vi "Perform Measurement - WaveformMode.vi"(8 "error in":errorcluster, 10 "Measure Call Context in":refnum<class "Measure Call Context.lvclass">, 11 "measurement configuration":T2={"Mode of operation"=enum."Power on the DUT", "Source voltage/current gain bandwidths"=[], "Source voltage/current compensation frequencies"=[], "Source voltage/current pole-zero ratios"=[], "Load voltage/current gain bandwidths"=[], "Load voltage/current compensation frequencies"=[], "Load voltage/current pole-zero ratios"=[], "Source enable/disable"=FALSE, "Load enable/disable"=FALSE, "Power ON/Source resource names"=[], "Load resource names"=[], "Power ON/Source voltage/current setpoints"=[], "Source source delays"=[], "Load voltage/current setpoints"=[], "Load source delays"=[], "Power ON/Source system configuration"=enum."Series", "Power ON/Source output function"=0, "Source voltage/current level range"=0.0, "Power ON/Source sense"=0, "Source limit symmetry"=enum."Symmetric", "Power ON/Source current/voltage limit range"=0.0, "Source current/voltage limit low"=0.0, "Source current/voltage limit high"=0.0, "Source aperture time"=0.0, "Source transient response"=0, "Load device voltage/current rating"=10.0, "Load system configuration"=enum."Series", "Load output function"=0, "Load voltage/current level range"=0.0, "Load sense"=0, "Load limit symmetry"=enum."Symmetric", "Load current/voltage limit range"=0.0, "Load current/voltage limit low"=0.0, "Load current/voltage limit high"=0.0, "Load aperture time"=0.0, "Load transient response"=0, "Measurement timeout"=1.0} {"Measurement timeout" format="%.3p"; "Load voltage/current setpoints" format="%#_6p"; "Load output function" items=["DC Voltage"=1006, "DC Current"=1007, "Pulse Voltage"=1049, "Pulse Current"=1050]; "Load sense" items=["Local"=1008, "Remote"=1009]; "Load transient response" items=["Slow"=1041, "Normal"=1038, "Fast"=1039, "Custom"=1042]; "Load current/voltage limit high" format="%#_6p"; "Load current/voltage limit low" format="%#_6p"; "Load current/voltage limit range" format="%#_6p"; "Load voltage/current level range" format="%#_6p"; "Power ON/Source voltage/current setpoints" format="%#_6p"; "Power ON/Source output function" items=["DC Voltage"=1006, "DC Current"=1007, "Pulse Voltage"=1049, "Pulse Current"=1050]; "Source aperture time" format="%#_6p"; "Power ON/Source sense" items=["DC Voltage"=1006, "DC Current"=1007, "Pulse Voltage"=1049, "Pulse Current"=1050]; "Source transient response" items=["Slow"=1041, "Normal"=1038, "Fast"=1039, "Custom"=1042]; "Source current/voltage limit high" format="%#_6p"; "Source current/voltage limit low" format="%#_6p"; "Power ON/Source current/voltage limit range" format="%#_6p"; "Source voltage/current level range" format="%#_6p"}) -> (0 "error out":errorcluster, 2 "Measure Call Context out":refnum<class "Measure Call Context.lvclass">, 3 "Measurement Results":T1)   [LabVIEW 2021, in "Waveform Mode_Channel Ganging.lvlib"]
uses:
  Waveform Mode_Channel Ganging.lvlib
  shared subVIs/ctl/NIDCPower_channel_ganging - ctl - channel mode.ctl
  shared subVIs/ctl/NIDCPower_channel_ganging - ctl - ganged config.ctl
  shared subVIs/ctl/NIDCPower_channel_ganging - ctl - ganged session.ctl
  Measurement Results.ctl
  shared/Single/controls/Initialize Resource Config-Single.ctl
  shared/Ganging/controls/Initialize Resource Config-Ganging.ctl
  <instrlib>/niDCPower/nidcpower.llb/niDCPower Wait For Event - Event.ctl
  shared/Common/controls/Start and Wait for Event.ctl
  shared/Ganging/controls/Abort Single Point-Ganging.ctl
  shared/Single/controls/Abort Single Point-Single.ctl
  Controls/Waveform Mode Measurement.ctl
  shared/Single/controls/Abort Sequence-Single.ctl
  shared/Ganging/controls/Abort Sequence-Ganging.ctl
  <vilib>/Plug-In SDKs/Measurements/Measure Call Context/Measure Call Context.lvclass
  Measurement Configuration.ctl
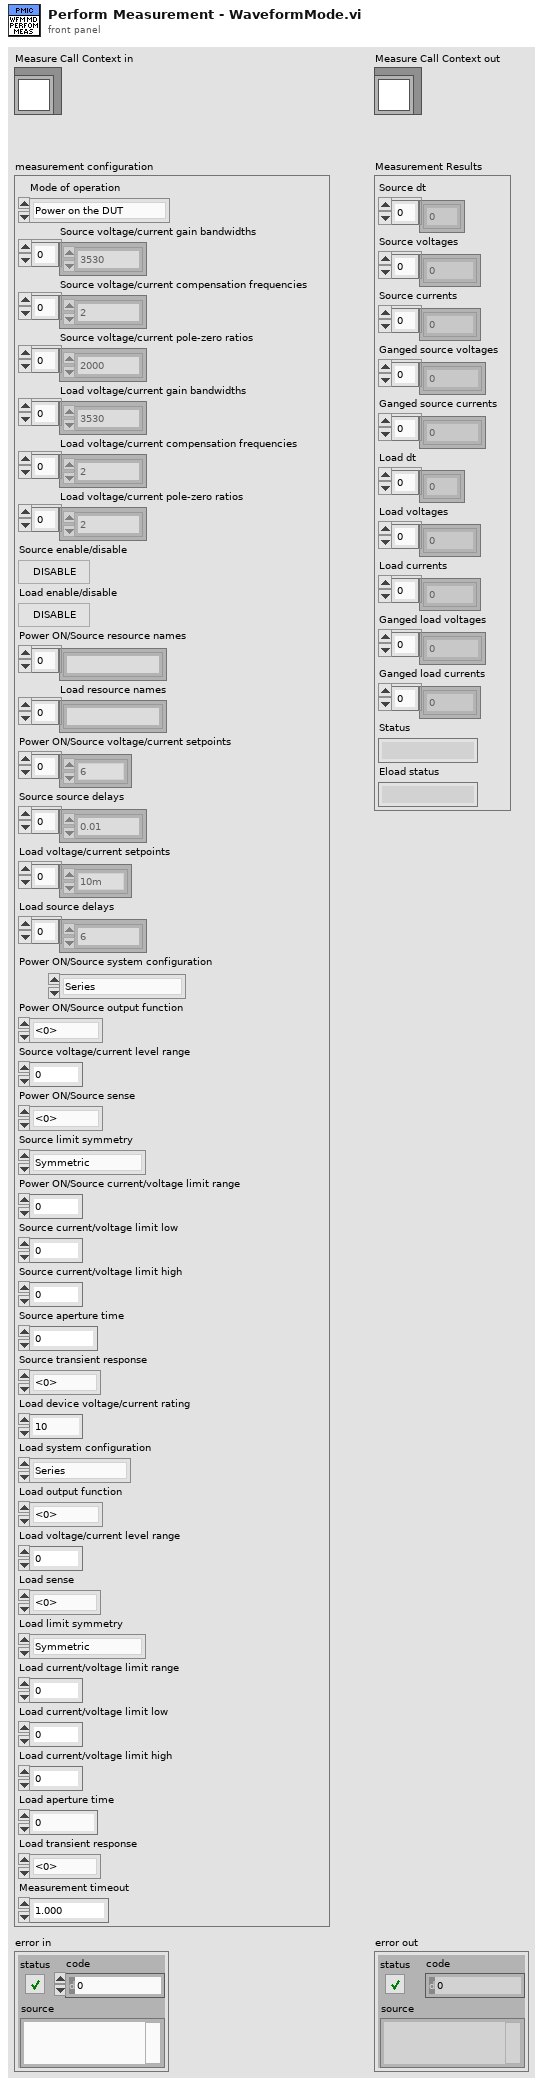
[diagram p1: front panel]
types:
  T1 = typedef "Waveform Mode_Channel Ganging.lvlib/Measurement Results.ctl" = cluster{"Source dt":dbl[], "Source voltages":dbl[], "Source currents":dbl[], "Ganged source voltages":dbl[], "Ganged source currents":dbl[], "Load dt":dbl[], "Load voltages":dbl[], "Load currents":dbl[], "Ganged load voltages":dbl[], "Ganged load currents":dbl[], "Status":string, "Eload status":string}
  T2 = typedef "Waveform Mode_Channel Ganging.lvlib/Measurement Configuration.ctl" = cluster{"Mode of operation":enum32{"Power on the DUT", "Perform measurement", "Power off the DUT"}, "Source voltage/current gain bandwidths":dbl[], "Source voltage/current compensation frequencies":dbl[], "Source voltage/current pole-zero ratios":dbl[], "Load voltage/current gain bandwidths":dbl[], "Load voltage/current compensation frequencies":dbl[], "Load voltage/current pole-zero ratios":dbl[], "Source enable/disable":bool, "Load enable/disable":bool, "Power ON/Source resource names":string[], "Load resource names":string[], "Power ON/Source voltage/current setpoints":dbl[], "Source source delays":dbl[], "Load voltage/current setpoints":dbl[], "Load source delays":dbl[], "Power ON/Source system configuration":enum32{"Series", "Parallel", "Manual"}, "Power ON/Source output function":i32, "Source voltage/current level range":dbl, "Power ON/Source sense":i32, "Source limit symmetry":enum32{"Symmetric", "Asymmetric"}, "Power ON/Source current/voltage limit range":dbl, "Source current/voltage limit low":dbl, "Source current/voltage limit high":dbl, "Source aperture time":dbl, "Source transient response":i32, "Load device voltage/current rating":dbl, "Load system configuration":enum32{"Series", "Parallel", "Manual"}, "Load output function":i32, "Load voltage/current level range":dbl, "Load sense":i32, "Load limit symmetry":enum32{"Symmetric", "Asymmetric"}, "Load current/voltage limit range":dbl, "Load current/voltage limit low":dbl, "Load current/voltage limit high":dbl, "Load aperture time":dbl, "Load transient response":i32, "Measurement timeout":dbl}
  T3 = typedef "Waveform Mode_Channel Ganging.lvlib/Waveform Mode Measurement.ctl" = cluster{"Source Ganged Session Out":T4, "Load Ganged Session Out":T4, "Source Measure Record Length":i32, "Load Measure Record Length":i32, "Source Sequence Name":string, "Load Sequence Name":string, "Source First Sequence Call":bool, "Load First Sequence Call":bool, "Measurement Results":T1, "No. of eload used":i32, "Measurement timeout":dbl, "Load Source ON/OFF":enum16{"SOURCE AND LOAD OFF", "SOURCE ON", "LOAD ON", "SOURCE AND LOAD ON"}, "Load session out":refnum<k15>, "Source session out":refnum<k15>, "Load channel name":string, "Source channel name":string, "Source ganged/single":bool, "Load ganged/single":bool, "Source Master/Single resource name":string, "Source Slave resource name":string[], "Load Master/Single resource name":string, "Load Slave resource name":string[]}
  T4 = typedef "NIDCPower_channel_ganging - ctl - ganged session.ctl" = cluster{"Ganged Config":T5, "Session List":refnum<k15>[], "Session Mode":T6[], "Channel":string[]}
  T5 = typedef "NIDCPower_channel_ganging - ctl - ganged config.ctl" = enum32{"Series", "Parallel", "Manual"}
  T6 = typedef "NIDCPower_channel_ganging - ctl - channel mode.ctl" = enum32{"Master", "Slave", "Slave - Inverted"}
  T7 = typedef "Initialize Resource Config-Ganging.ctl" = cluster{"Master resource name ":string, "Slave resource names":string[], "System configuration":enum32{"Series", "Parallel", "Manual"}, "Voltage/current level":dbl, "Voltage/current level range":dbl, "Limit symmetry":enum32{"Symmetric", "Asymmetric"}, "Voltage/current limit range":dbl, "Voltage/current limit low":dbl, "Voltage/current limit high":dbl, "Output function":i32, "Sense":i32, "Transient response":i32, "Voltage/current gain bandwith":dbl, "Voltage/current compensation frequency":dbl, "Voltage/current pole-zero ratio":dbl, "DUT set-up time":dbl}
  T8 = typedef "Initialize Resource Config-Single.ctl" = cluster{"Resource name":string, "Voltage/current level":dbl, "Voltage/current level range":dbl, "Voltage/current limit range":dbl, "Voltage/current limit low":dbl, "Voltage/current limit high":dbl, "Output function":i32, "Sense":i32, "Transient response":i32, "Voltage/current gain bandwidth":dbl, "Voltage/current compensation frequency":dbl, "Voltage/current pole-zero ratio":dbl, "DUT set-up time":dbl, "Limit symmetry":enum32{"Symmetric", "Asymmetric"}}
  T9 = typedef "Start and Wait for Event.ctl" = cluster{"Source Ganged Session Out":T4, "Load Ganged Session Out":T4, "Source session out":refnum<k15>, "Load session out":refnum<k15>, "event":T10, "Source channel name":string, "Load channel name":string, "Load Source ON/OFF":enum16{"SOURCE AND LOAD OFF", "SOURCE ON", "LOAD ON", "SOURCE AND LOAD ON"}, "Load ganged/single":bool, "Source ganged/single":bool}
  T10 = typedef "niDCPower Wait For Event - Event.ctl" = i32
  T11 = typedef "Abort Single Point-Ganging.ctl" = cluster{"Ganged Session in":cluster{"Ganged Config":T5, "Session List":refnum<k15>[], "Session Mode":T6[], "Channel":string[]}}
  T12 = typedef "Abort Single Point-Single.ctl" = cluster{"Resource out":refnum<k15>, "Resource channel name":string}
  T13 = typedef "Abort Sequence-Ganging.ctl" = cluster{"Ganged Session Out":cluster{"Ganged Config":T5, "Session List":refnum<k15>[], "Session Mode":T6[], "Channel":string[]}, "Sequence name":string}
  T14 = typedef "Abort Sequence-Single.ctl" = cluster{"Resource out":refnum<k15>, "Resource channel name":string, "Source sequence name":string}
  T15 = enum32{"Power on the DUT", "Perform measurement", "Power off the DUT"}
  T16 = enum16{"SOURCE AND LOAD OFF", "SOURCE ON", "LOAD ON", "SOURCE AND LOAD ON"}
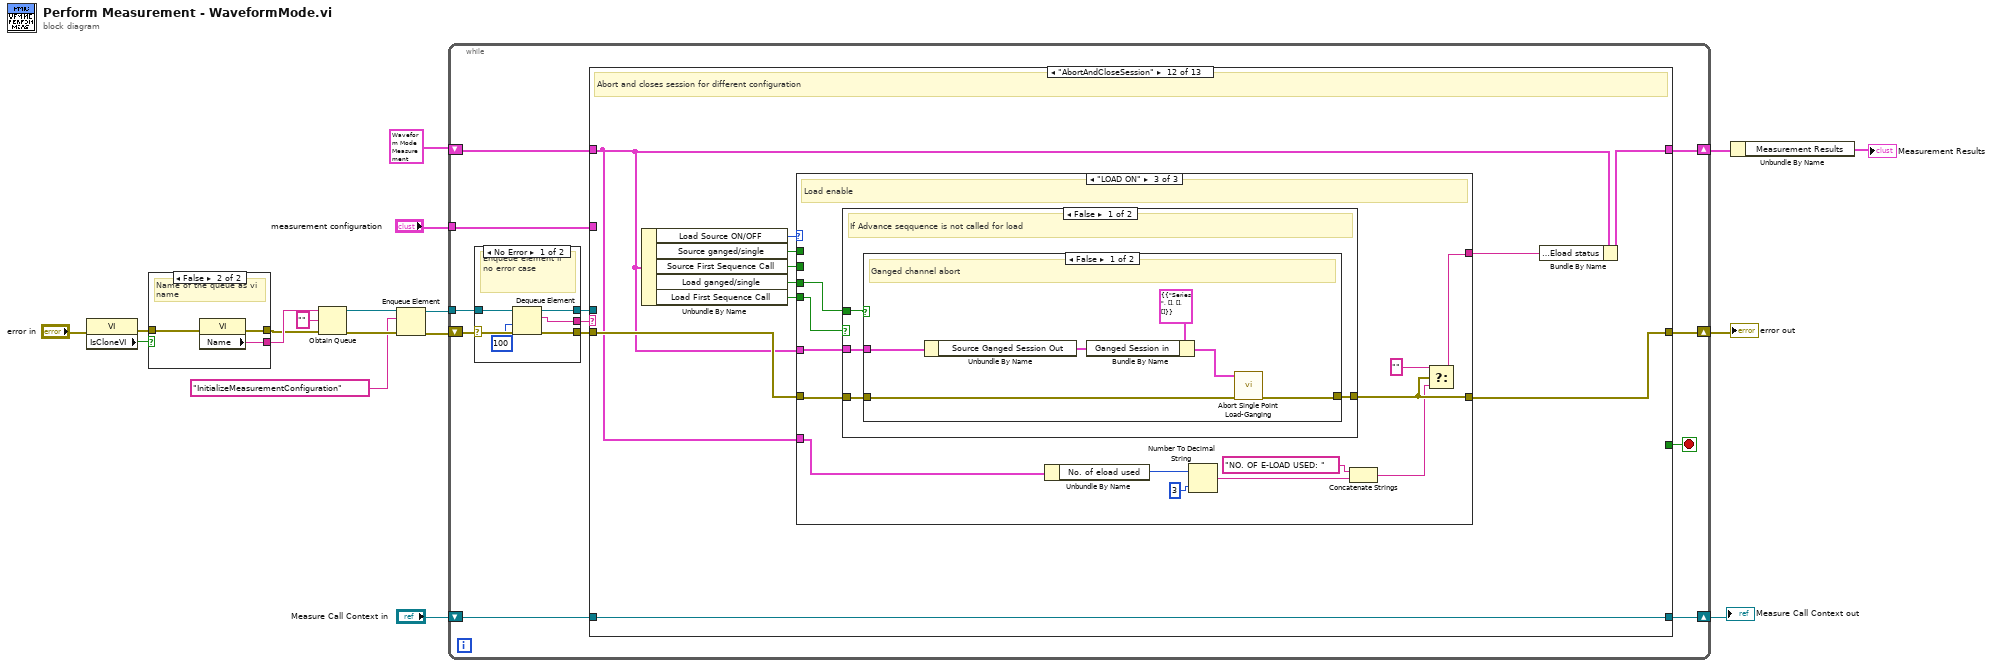
[diagram p0: block diagram]
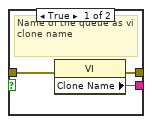
[diagram p2: hidden frame]
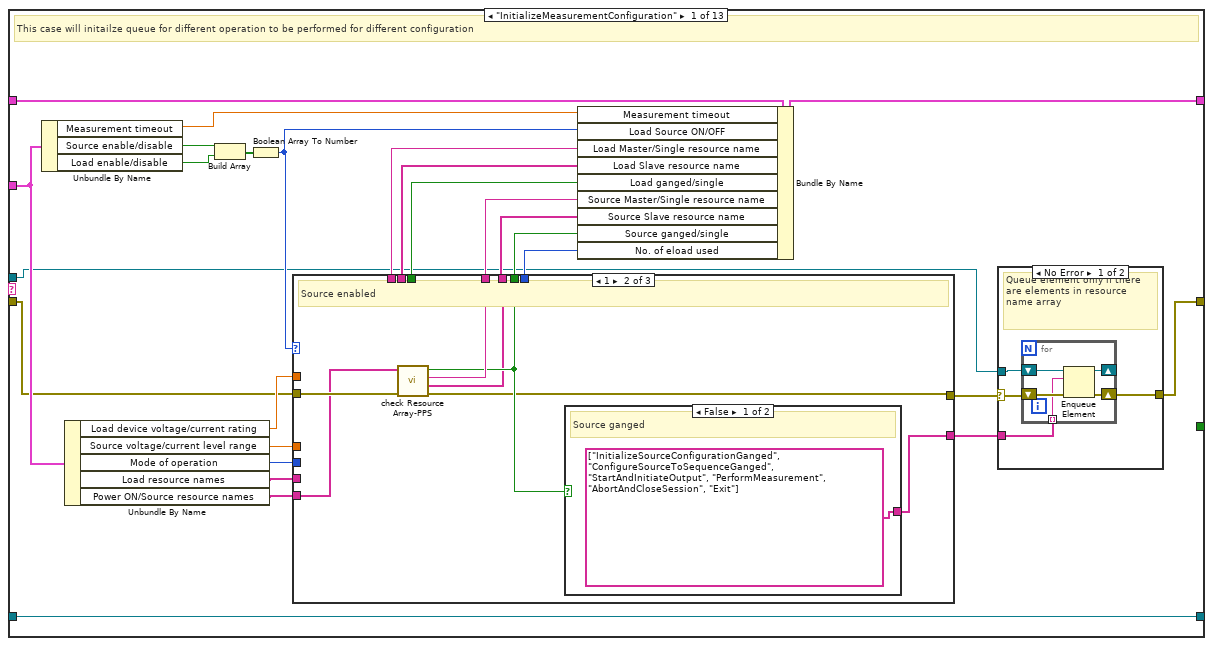
[diagram p3: hidden frame]
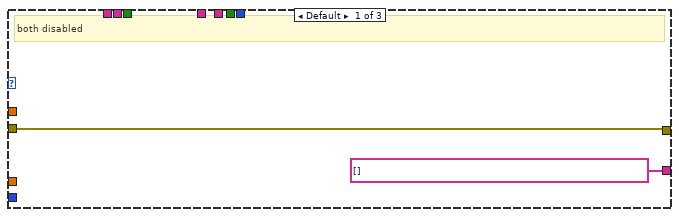
[diagram p5: hidden frame]
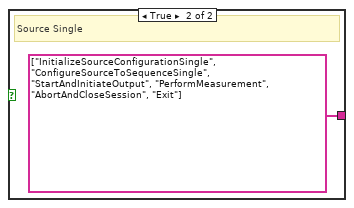
[diagram p6: hidden frame]
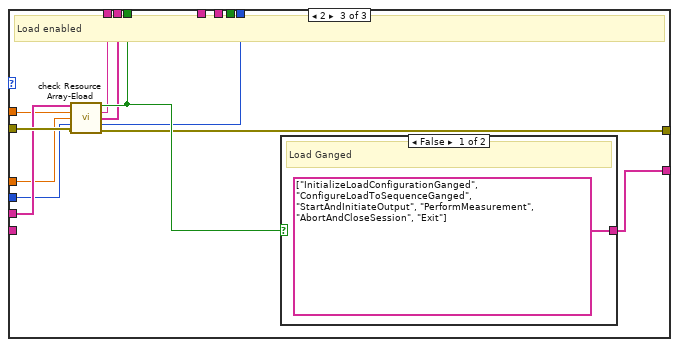
[diagram p7: hidden frame]
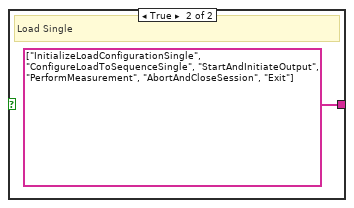
[diagram p8: hidden frame]
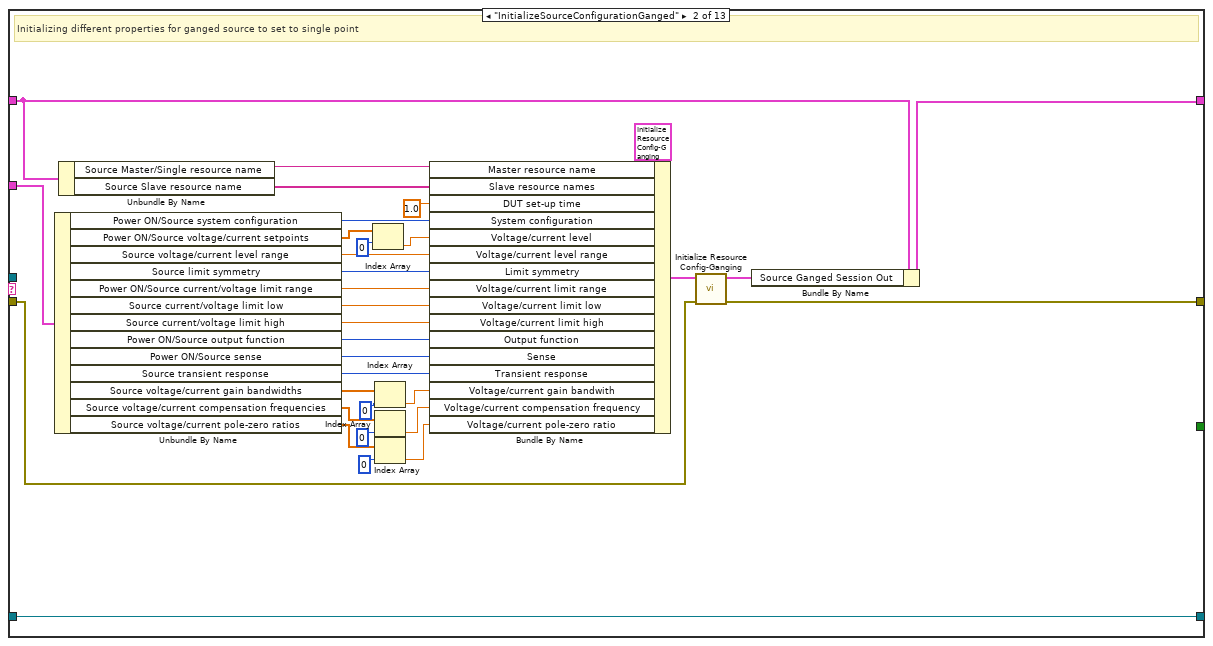
[diagram p9: hidden frame]
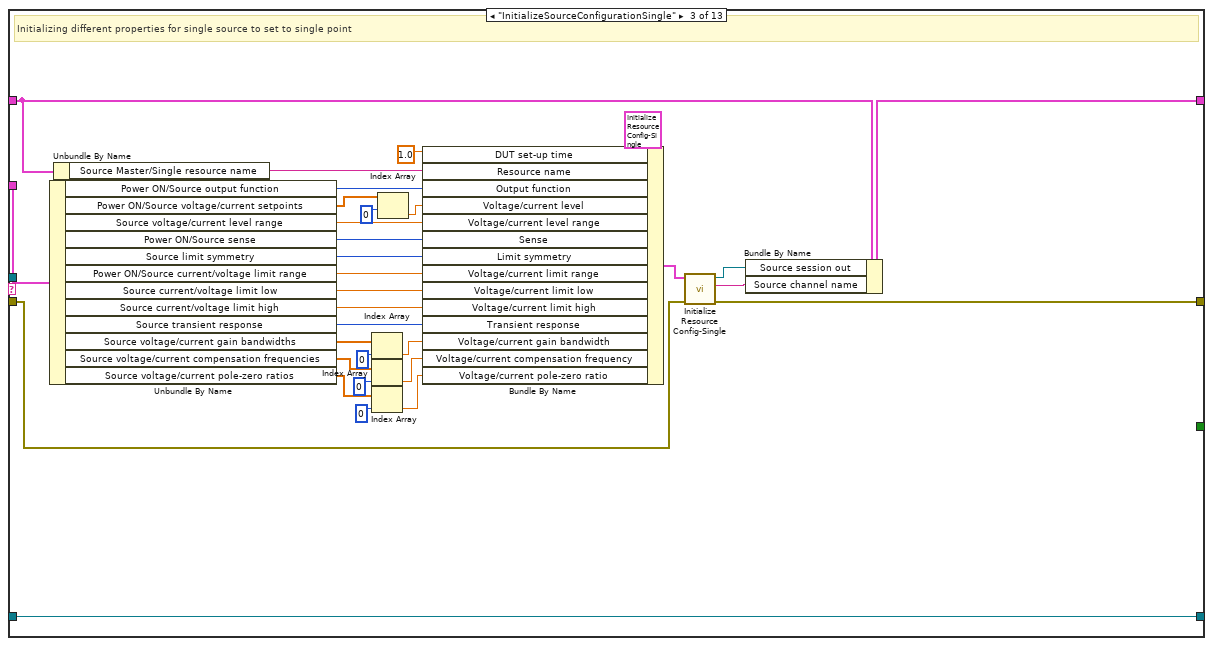
[diagram p10: hidden frame]
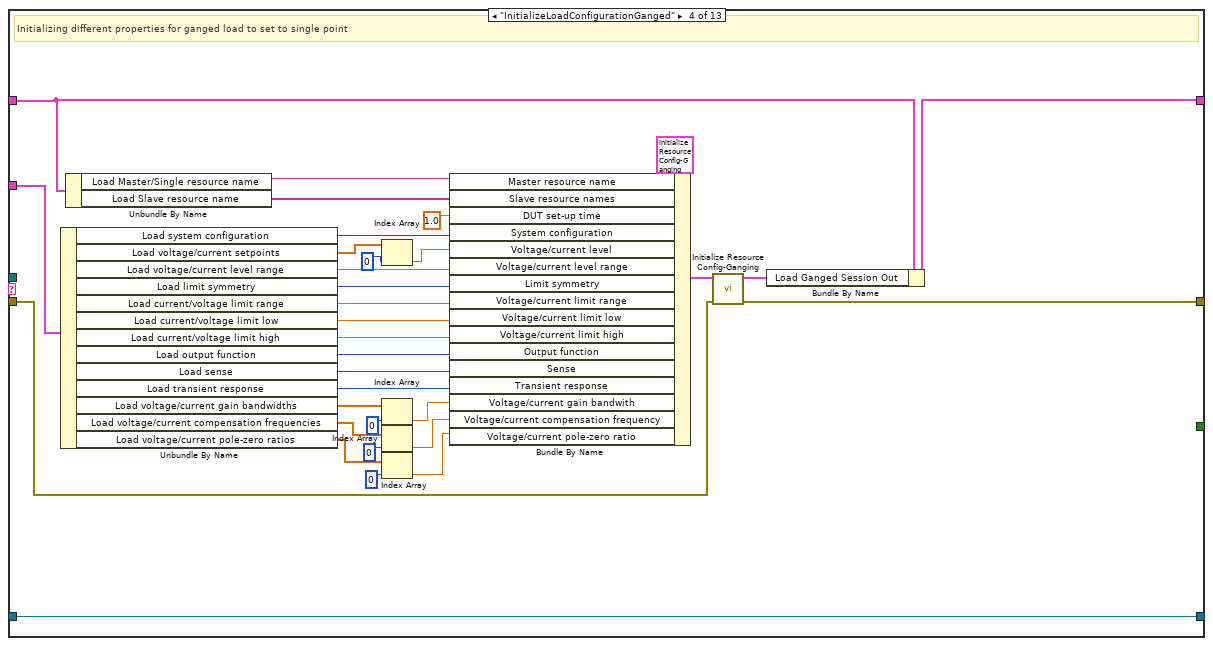
[diagram p11: hidden frame]
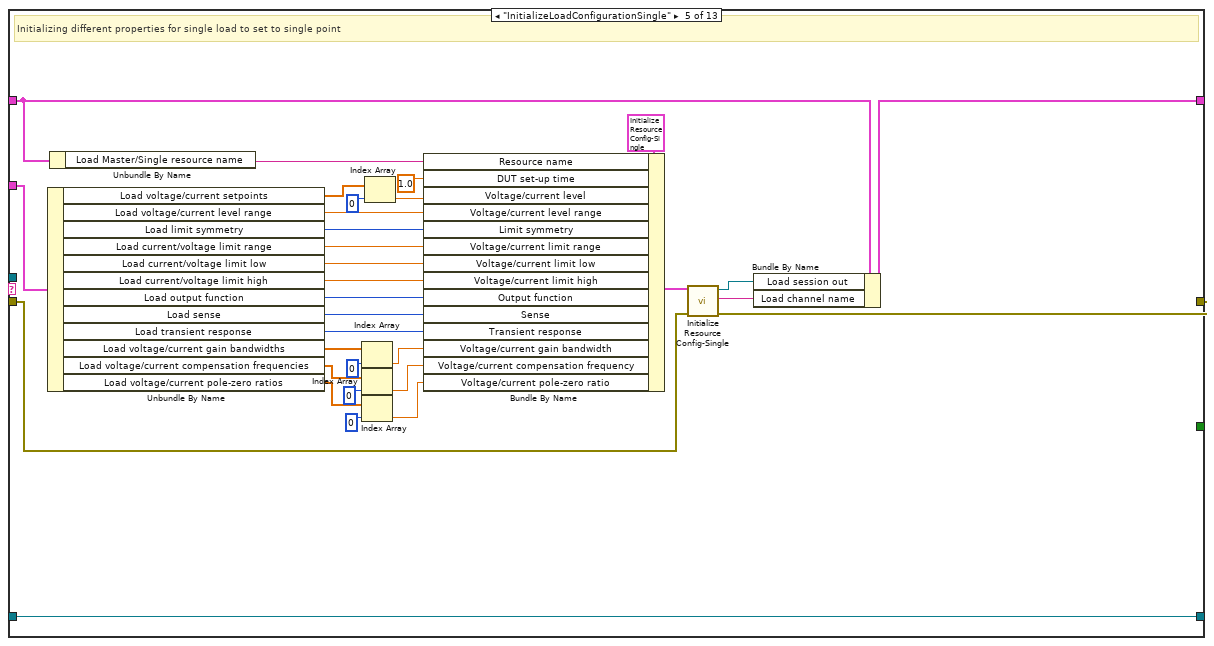
[diagram p12: hidden frame]
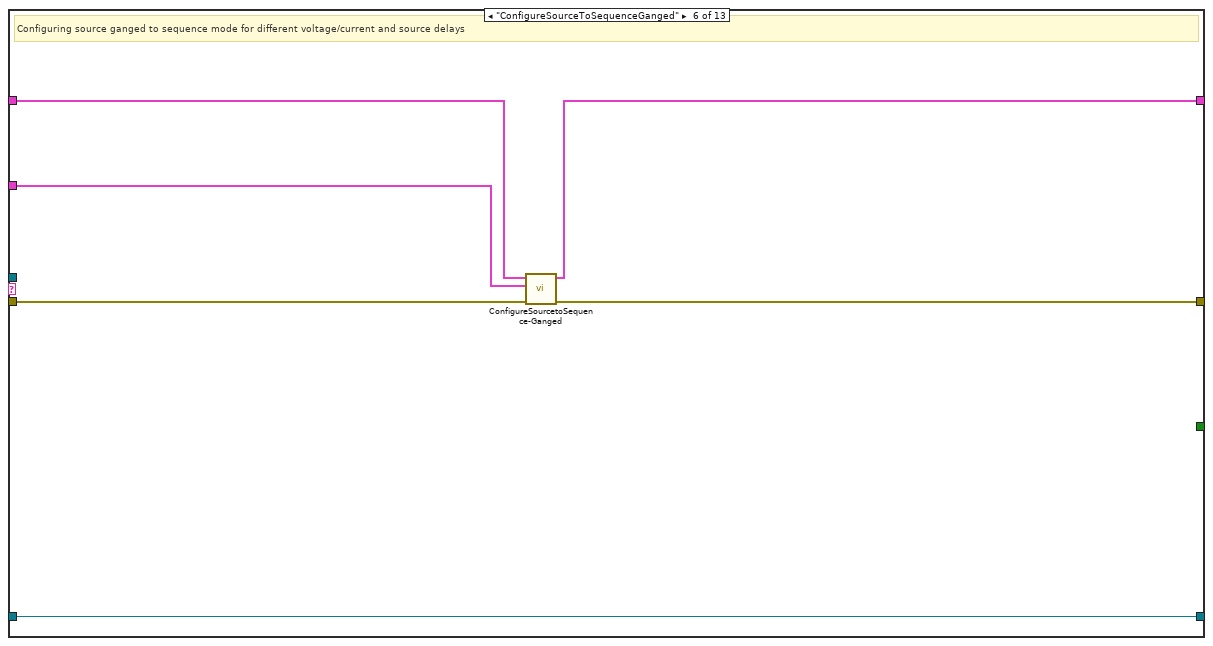
[diagram p13: hidden frame]
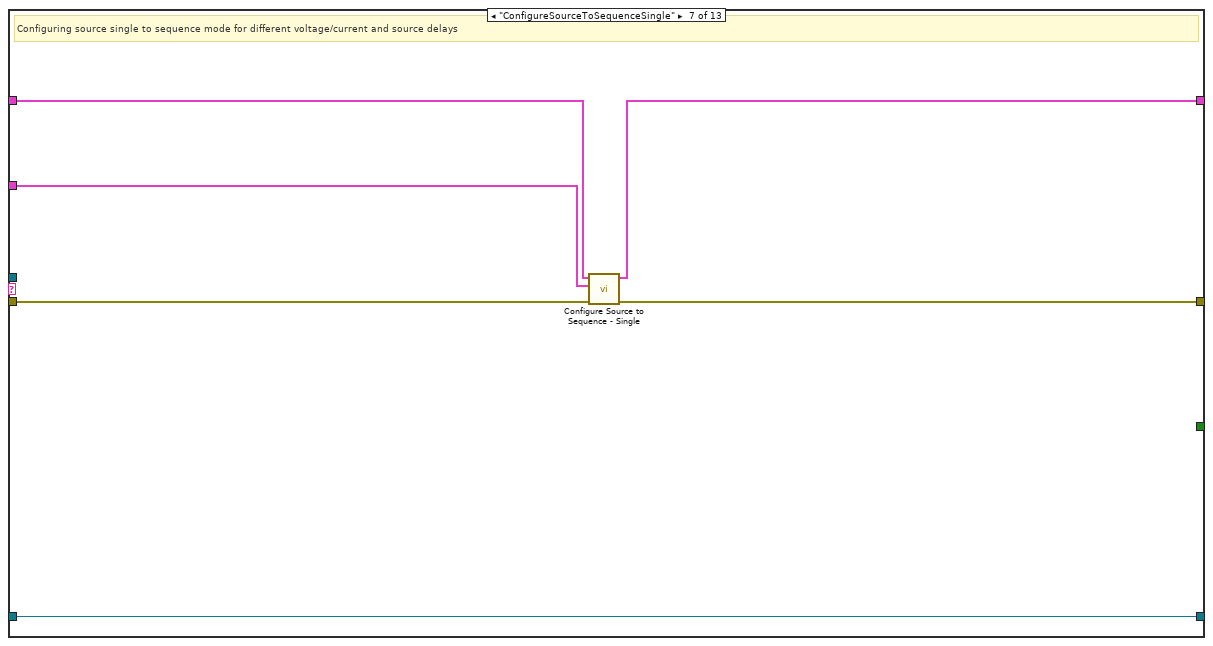
[diagram p14: hidden frame]
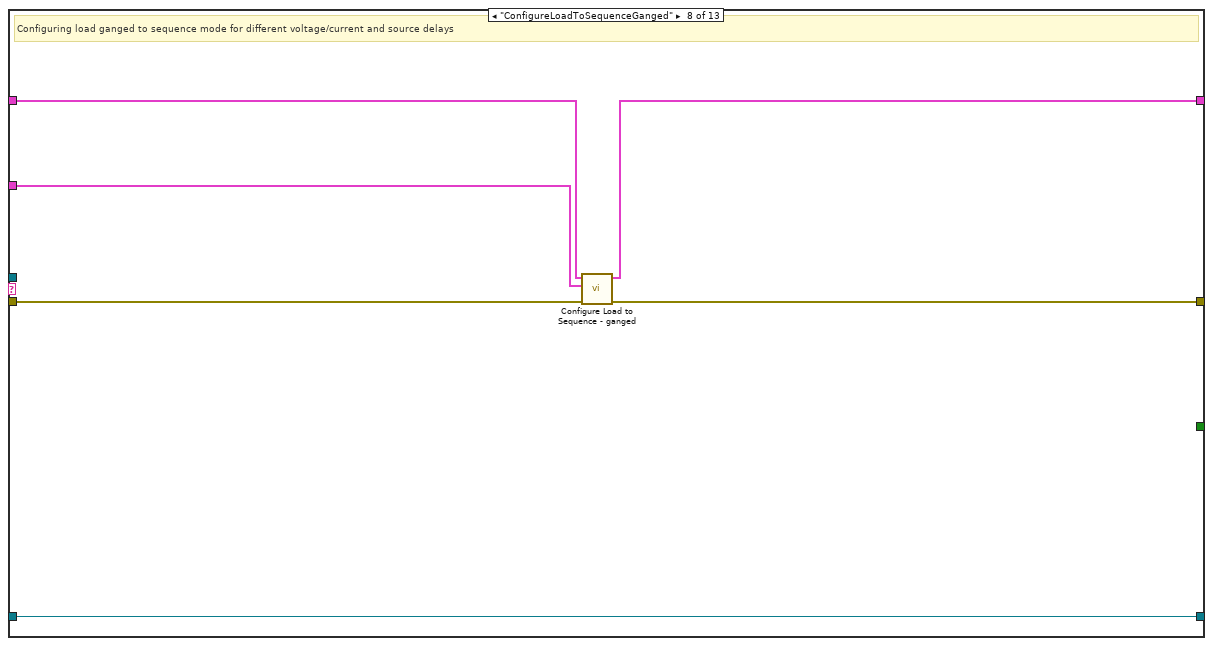
[diagram p15: hidden frame]
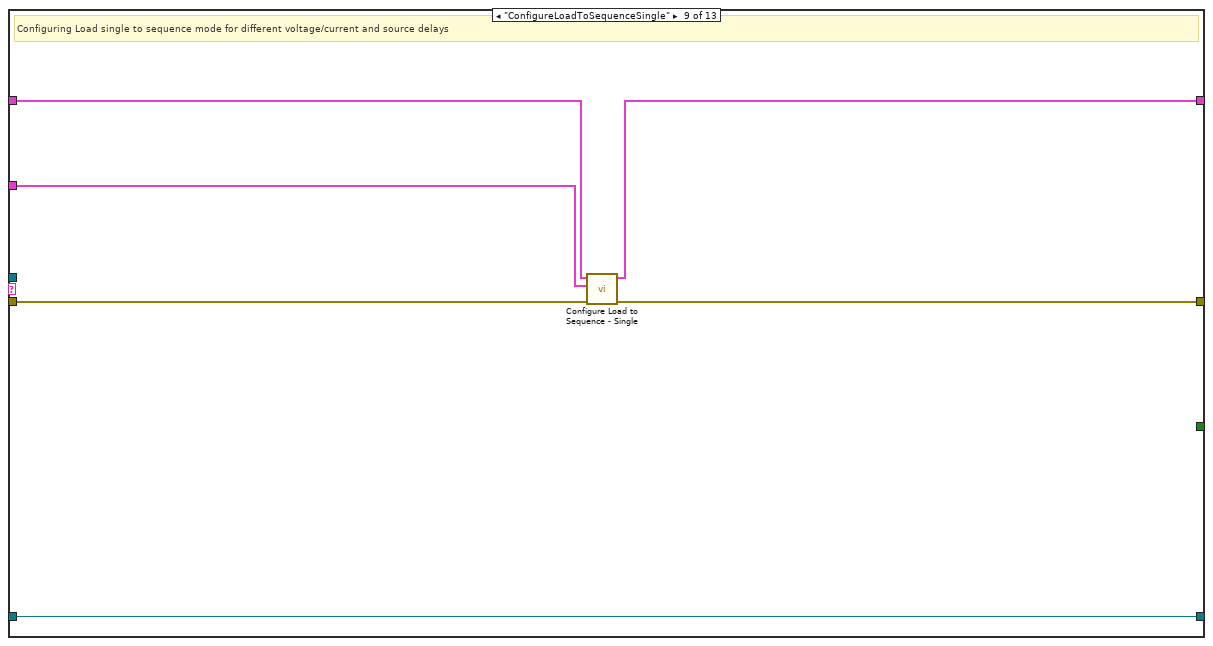
[diagram p16: hidden frame]
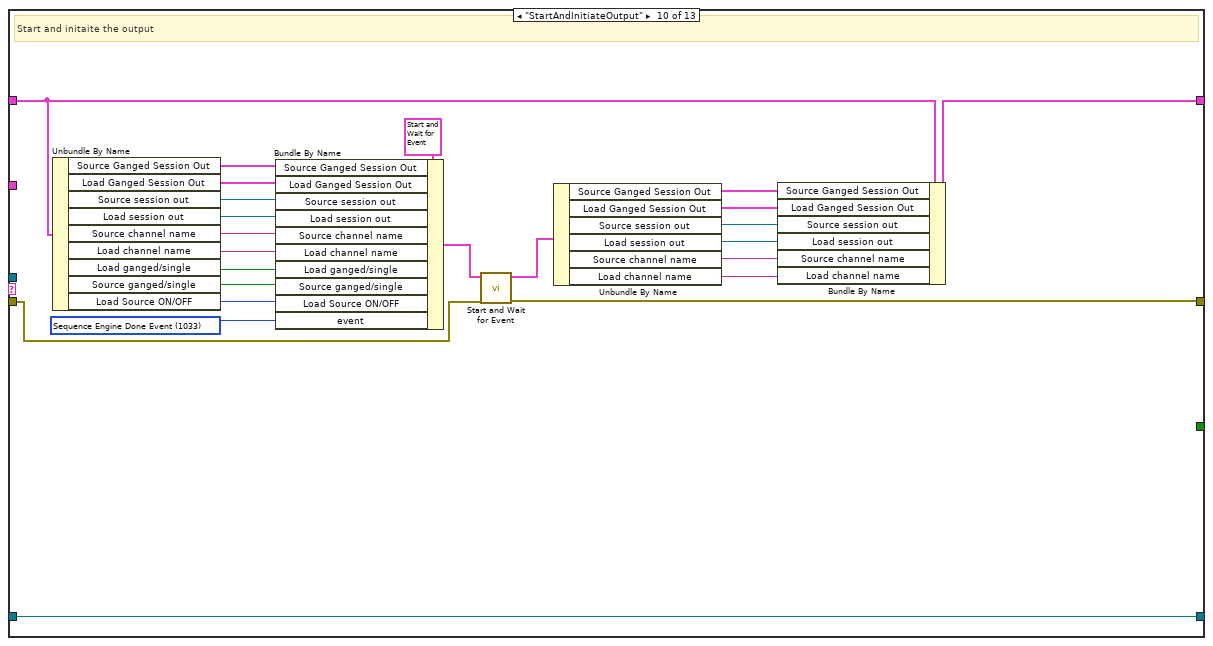
[diagram p17: hidden frame]
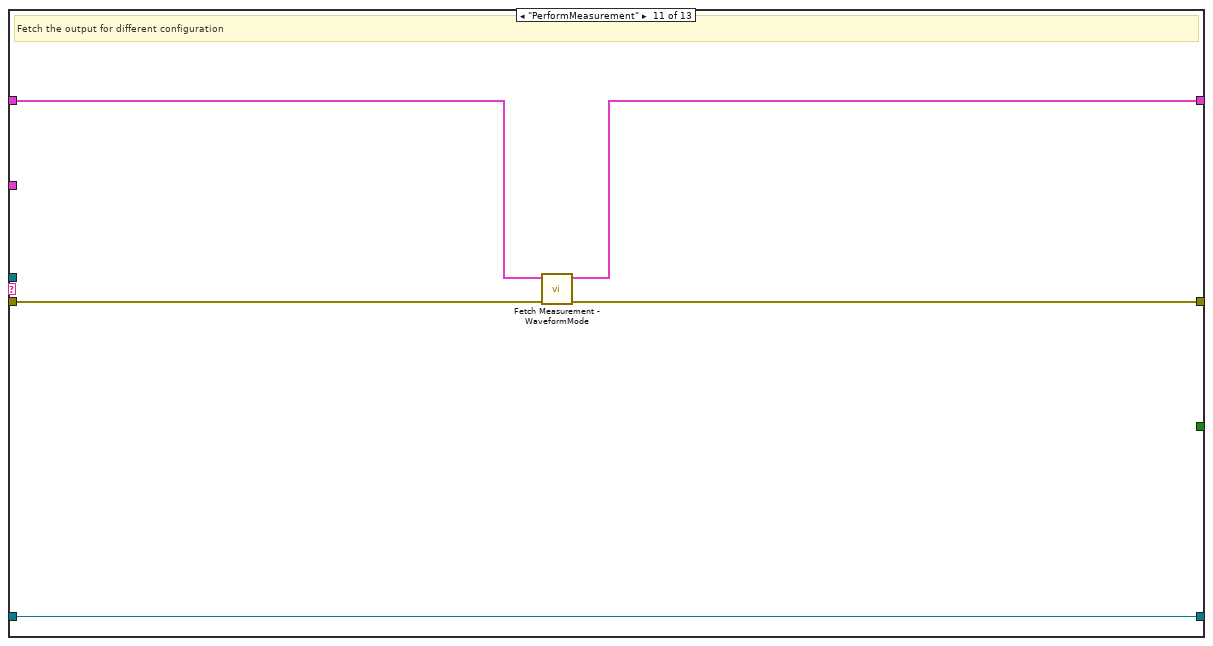
[diagram p18: hidden frame]
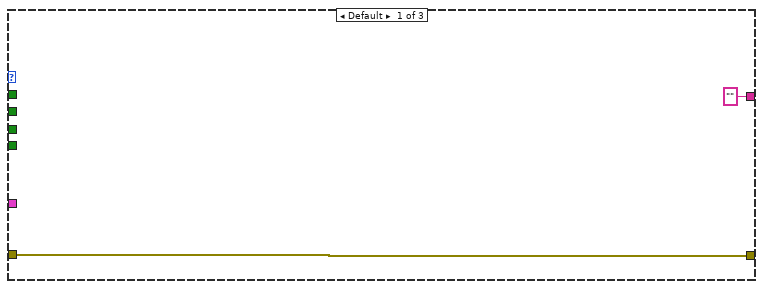
[diagram p19: hidden frame]
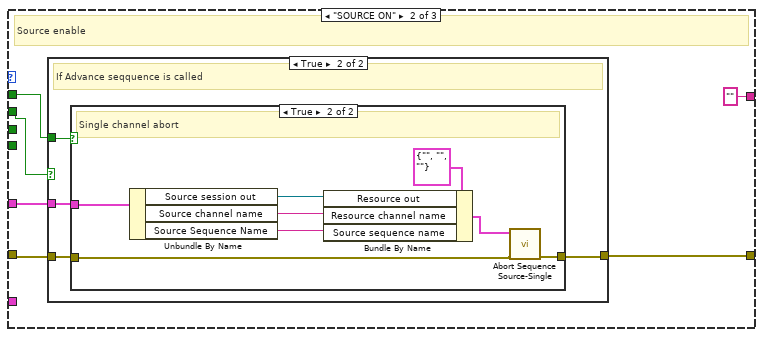
[diagram p20: hidden frame]
diagram:
  n1 = property class="VI"(error in="error in") -> (error out=w10:errorcluster, "IsCloneVI"=w9:bool)  [unwired: 1 in, 1 out]
  n2 = case shown="False" w9 {
    tunnel: [w21 w24] -> w11
    tunnel: [w20 w23] -> w12
    tunnel: w10 -> [w19 w22]
    frame True {
      # "Name of the queue as vi clone name"
      n3 = property class="VI"(error in=w19) -> (error out=w21:errorcluster, "Clone Name"=w20:string)  [unwired: 1 in, 1 out]
    }
    frame False {
      # "Name of the queue as vi name"
      n4 = property class="VI"(error in=w22) -> (error out=w24:errorcluster, "Name"=w23:string)  [unwired: 1 in, 1 out]
    }
  }
  n5 = Obtain Queue(name (unnamed)=w12, element data type="", error in (no error)=w11) -> (queue out=w7:refnum<queue>, error out=w8:errorcluster)  [unwired: 2 in, 1 out]
  n6 = Enqueue Element(queue=w7, element="InitializeMeasurementConfiguration" ("Step sequence"), error in (no error)=w8) -> (queue out=w4:refnum<queue>, error out=w3:errorcluster)  [unwired: 1 in, 1 out]
  n7 = while {
    tunnel: w4 -> [w36]
    shift-right: [w30] -> w15
    shift-left: T3 {"Source Ganged Session Out"={"Ganged Config"=enum."Series", "Session List"=[], "Session Mode"=[], "Channel"=[]}, "Load Ganged Session Out"={"Ganged Config"=enum."Series", "Session List"=[], "Session Mode"=[], "Channel"=[]}, "Source Measure Record Length"=0, "Load Measure Record Length"=0, "Source Sequence Name"="", "Load Sequence Name"="", "Source First Sequence Call"=FALSE, "Load First Sequence Call"=FALSE, "Measurement Results"={"Source dt"=[], "Source voltages"=[], "Source currents"=[], "Ganged source voltages"=[], "Ganged source currents"=[0.0], "Load dt"=[], "Load voltages"=[], "Load currents"=[], "Ganged load voltages"=[], "Ganged load currents"=[], "Status"="", "Eload status"=""}, "No. of eload used"=0, "Measurement timeout"=0.0, "Load Source ON/OFF"=enum."SOURCE AND LOAD ON", "Load session out"="", "Source session out"="", "Load channel name"="", "Source channel name"="", "Source ganged/single"=FALSE, "Load ganged/single"=FALSE, "Source Master/Single resource name"="", "Source Slave resource name"=[], "Load Master/Single resource name"="", "Load Slave resource name"=[]} -> [w31]
    shift-right: [w29] -> w18
    shift-left: w3 -> [w35]
    shift-right: [w25] -> w14
    shift-left: "Measure Call Context in" -> [w26]
    tunnel: "measurement configuration" -> [w27]
    stop <- w28 stop-if-true
    n8 = case shown="No Error" w35 {
      selector: w35 -> [w391 w395]
      tunnel: w36 -> [w393 w394]
      tunnel: [w392 "Exit" ("t")] -> w34
      tunnel: [w390 w395] -> w32
      tunnel: [w388 w394] -> w33
      frame No Error {
        # "Enqueue element if  no error case"
        n9 = Dequeue Element(queue=w393, timeout in ms (-1)=100, error in (no error)=w391) -> (queue out=w388:refnum<queue>, element=w392:string, error out=w390:errorcluster)  [unwired: 1 out]
      }
      frame Error {
        # "Don't Enqueue element if error case"
      }
    }
    n10 = case shown="\"AbortAndCloseSession\"" w34 {
      tunnel: w33 -> [w42 _ _ _ _ _ _ _ _ _ _ _ _]
      tunnel: w32 -> [w41 w115 w147 w178 w211 w232 w238 w244 w250 w256 w279 w282 w386]
      tunnel: w31 -> [w44 w100 w133 w180 w212 w229 w236 w241 w248 w254 w276 w281 w385]
      tunnel: [w40 w99 w132 w164 w209 w231 w235 w243 w245 w253 w278 w286 w385] -> w30
      tunnel: [w39 w98 w131 w163 w196 w228 w234 w240 w247 w255 w277 w287 w386] -> w29
      tunnel: [_ _ _ _ _ _ _ _ _ _ _ _ TRUE] -> w28
      tunnel: w27 -> [w43 w114 w146 w179 w213 w230 w237 w242 w249 _ _ _ _]
      tunnel: w26 -> [w38 w97 w130 w162 w195 w227 w233 w239 w246 w251 w275 w285 w384]
      tunnel: [w38 w97 w130 w162 w195 w227 w233 w239 w246 w251 w275 w285 w384] -> w25
      frame "InitializeMeasurementConfiguration" {
        # "This case will initailze queue for different operation to be performed for different configuration"
        n11 = Unbundle By Name(w43) -> ("Measurement timeout"=w46:dbl, "Source enable/disable"=w52:bool, "Load enable/disable"=w51:bool)
        n12 = Unbundle By Name(w43) -> ("Load device voltage/current rating"=w61:dbl, "Source voltage/current level range"=w62:dbl, "Mode of operation"=w37:T15, "Load resource names"=w53:string[], "Power ON/Source resource names"=w54:string[])
        n13 = Build Array(w52, w51) -> (w50:bool[])
        n14 = Boolean Array To Number(Boolean array=w50) -> (number=w47:u32)
        n15 = case shown="1" w47 {
          tunnel: w41 -> [w73 w81 w94]
          tunnel: [w73 w76 w88] -> w45
          tunnel: w53 -> [_ _ w93]
          tunnel: w54 -> [_ w80 _]
          tunnel: [_ _ w91] -> w55
          tunnel: [_ _ w90] -> w56
          tunnel: [_ w79 _] -> w57
          tunnel: [_ w77 _] -> w58
          tunnel: [_ _ w92] -> w59
          tunnel: [_ w78 _] -> w60
          tunnel: w61 -> [_ _ w89]
          tunnel: w62 -> [_ _ w85]
          tunnel: [string[] [] ("Step sequence") w75 w87] -> w49
          tunnel: [_ _ w86] -> w48
          tunnel: w37 -> [_ _ w84]
          frame Default {
            # "both disabled"
          }
          frame 1 {
            # "Source enabled"
            n16 = call "check Resource Array-PPS.vi"("error in"=w81, "Resource names"=w80) -> ("error out"=w76:errorcluster, "Slave resource names"=w77:string[], "Single/Master resouce names"=w79:string, "Single or ganged configuration"=w78:bool)  [unwired: 6 in]
            n17 = case shown="False" w78 {
              tunnel: [string[] ["InitializeSourceConfigurationGanged", "ConfigureSourceToSequenceGanged", "StartAndInitiateOutput", "PerformMeasurement", "AbortAndCloseSession", "Exit"] ("Step sequence") string[] ["InitializeSourceConfigurationSingle", "ConfigureSourceToSequenceSingle", "StartAndInitiateOutput", "PerformMeasurement", "AbortAndCloseSession", "Exit"] ("Step sequence")] -> w75
              frame False {
                # "Source ganged"
              }
              frame True {
                # "Source Single"
              }
            }
          }
          frame 2 {
            # "Load enabled"
            n18 = call "check Resource Array-Eload.vi"("Resource names"=w93, "Device current rating"=w89, "Expected current level"=w85, "Mode of operation"=w84, "error in"=w94) -> ("Single or ganged configuration"=w92:bool, "Single/Master resouce name"=w91:string, "Slave resource names"=w90:string[], "Number of devices used"=w86:i32, "error out"=w88:errorcluster)  [unwired: 6 in]
            n19 = case shown="False" w92 {
              tunnel: [string[] ["InitializeLoadConfigurationGanged", "ConfigureLoadToSequenceGanged", "StartAndInitiateOutput", "PerformMeasurement", "AbortAndCloseSession", "Exit"] ("Step sequence") string[] ["InitializeLoadConfigurationSingle", "ConfigureLoadToSequenceSingle", "StartAndInitiateOutput", "PerformMeasurement", "AbortAndCloseSession", "Exit"] ("Step sequence")] -> w87
              frame False {
                # "Load Ganged"
              }
              frame True {
                # "Load Single"
              }
            }
          }
        }
        n20 = Bundle By Name(cluster=w44, "Measurement timeout"=w46, "Load Source ON/OFF"=w47, "Load Master/Single resource name"=w55, "Load Slave resource name"=w56, "Load ganged/single"=w59, "Source Master/Single resource name"=w57, "Source Slave resource name"=w58, "Source ganged/single"=w60, "No. of eload used"=w48) -> (w40:T3)
        n21 = case shown="No Error" w45 {
          selector: w45 -> [w63 w72]
          tunnel: w49 -> [w66 _]
          tunnel: [w65 w72] -> w39
          tunnel: w42 -> [w64 _]
          frame No Error {
            # "Queue element only if there are elements in resource name array"
            n22 = for {
              shift-right: [w69] -> _
              shift-left: w64 -> [w71]
              shift-right: [w68] -> w65
              shift-left: w63 -> [w70]
              tunnel: w66 -> [w67] mode=indexing
              n23 = Enqueue Element(queue=w71, element=w67, error in (no error)=w70) -> (queue out=w69:refnum<queue>, error out=w68:errorcluster)  [unwired: 1 in, 1 out]
            }
          }
          frame Error {
            # "If error directly goes to exit case"
          }
        }
      }
      frame "InitializeSourceConfigurationGanged" {
        # "Initializing different properties for ganged source to set to single point"
        n24 = Unbundle By Name(w114) -> ("Power ON/Source system configuration"=w125:enum32{"Series", "Parallel", "Manual"}, "Power ON/Source voltage/current setpoints"=w102:dbl[], "Source voltage/current level range"=w124:dbl, "Source limit symmetry"=w123:enum32{"Symmetric", "Asymmetric"}, "Power ON/Source current/voltage limit range"=w117:dbl, "Source current/voltage limit low"=w118:dbl, "Source current/voltage limit high"=w119:dbl, "Power ON/Source output function"=w120:i32, "Power ON/Source sense"=w121:i32, "Source transient response"=w122:i32, "Source voltage/current gain bandwidths"=w109:dbl[], "Source voltage/current compensation frequencies"=w108:dbl[], "Source voltage/current pole-zero ratios"=w107:dbl[])
        n25 = Unbundle By Name(w100) -> ("Source Master/Single resource name"=w127:string, "Source Slave resource name"=w126:string[])
        n26 = Index Array(array=w102, index=0) -> (element=w101:dbl)
        n27 = Index Array(array=w109, index=0) -> (element=w106:dbl)
        n28 = Index Array(array=w108, index=0) -> (element=w105:dbl)
        n29 = Index Array(array=w107, index=0) -> (element=w104:dbl)
        n30 = Bundle By Name(cluster=T7 {"Master resource name "="", "Slave resource names"=[], "System configuration"=enum."Parallel", "Voltage/current level"=0.0, "Voltage/current level range"=0.0, "Limit symmetry"=enum."Symmetric", "Voltage/current limit range"=0.0, "Voltage/current limit low"=0.0, "Voltage/current limit high"=inf, "Output function"=1007, "Sense"=1009, "Transient response"=1038, "Voltage/current gain bandwith"=0.0, "Voltage/current compensation frequency"=0.0, "Voltage/current pole-zero ratio"=0.0, "DUT set-up time"=0.0} ("Initialize Resource Config - Ganging"), "Master resource name"=w127, "Slave resource names"=w126, "DUT set-up time"=1.0, "System configuration"=w125, "Voltage/current level"=w101, "Voltage/current level range"=w124, "Limit symmetry"=w123, "Voltage/current limit range"=w117, "Voltage/current limit low"=w118, "Voltage/current limit high"=w119, "Output function"=w120, "Sense"=w121, "Transient response"=w122, "Voltage/current gain bandwith"=w106, "Voltage/current compensation frequency"=w105, "Voltage/current pole-zero ratio"=w104) -> (w129:T7)
        n31 = call "Initialize Resource Config-Ganging.vi"("error in"=w115, "Initialize Resource Config - Ganging"=w129) -> ("error out"=w98:errorcluster, "Ganged Session Out"=w116:T4)  [unwired: 8 in]
        n32 = Bundle By Name(cluster=w100, "Source Ganged Session Out"=w116) -> (w99:T3)
      }
      frame "InitializeSourceConfigurationSingle" {
        # "Initializing different properties for single source to set to single point"
        n33 = Unbundle By Name(w146) -> ("Power ON/Source output function"=w161:i32, "Power ON/Source voltage/current setpoints"=w145:dbl[], "Source voltage/current level range"=w160:dbl, "Power ON/Source sense"=w159:i32, "Source limit symmetry"=w158:enum32{"Symmetric", "Asymmetric"}, "Power ON/Source current/voltage limit range"=w157:dbl, "Source current/voltage limit low"=w156:dbl, "Source current/voltage limit high"=w155:dbl, "Source transient response"=w154:i32, "Source voltage/current gain bandwidths"=w139:dbl[], "Source voltage/current compensation frequencies"=w142:dbl[], "Source voltage/current pole-zero ratios"=w140:dbl[])
        n34 = Unbundle By Name(w133) -> ("Source Master/Single resource name"=w151:string)
        n35 = Index Array(array=w139, index=0) -> (element=w138:dbl)
        n36 = Index Array(array=w142, index=0) -> (element=w137:dbl)
        n37 = Index Array(array=w140, index=0) -> (element=w141:dbl)
        n38 = Index Array(array=w145, index=0) -> (element=w143:dbl)
        n39 = Bundle By Name(cluster=T8 {"Resource name"="", "Voltage/current level"=0.0, "Voltage/current level range"=0.0, "Voltage/current limit range"=0.0, "Voltage/current limit low"=0.0, "Voltage/current limit high"=inf, "Output function"=1007, "Sense"=1009, "Transient response"=1038, "Voltage/current gain bandwidth"=0.0, "Voltage/current compensation frequency"=0.0, "Voltage/current pole-zero ratio"=0.0, "DUT set-up time"=0.0, "Limit symmetry"=enum."Symmetric"} ("Initialize Resource Config - Single"), "DUT set-up time"=1.0, "Resource name"=w151, "Output function"=w161, "Voltage/current level"=w143, "Voltage/current level range"=w160, "Sense"=w159, "Limit symmetry"=w158, "Voltage/current limit range"=w157, "Voltage/current limit low"=w156, "Voltage/current limit high"=w155, "Transient response"=w154, "Voltage/current gain bandwidth"=w138, "Voltage/current compensation frequency"=w137, "Voltage/current pole-zero ratio"=w141) -> (w152:T8)
        n40 = call "Initialize Resource Config-Single.vi"("error in"=w147, "Initialize resource Config - Single"=w152) -> ("error out"=w131:errorcluster, "channel name"=w150:string, "instrument handle out"=w149:refnum<k15>)  [unwired: 7 in]
        n41 = Bundle By Name(cluster=w133, "Source session out"=w149, "Source channel name"=w150) -> (w132:T3)
      }
      frame "InitializeLoadConfigurationGanged" {
        # "Initializing different properties for ganged load to set to single point"
        n42 = Unbundle By Name(w179) -> ("Load system configuration"=w189:enum32{"Series", "Parallel", "Manual"}, "Load voltage/current setpoints"=w167:dbl[], "Load voltage/current level range"=w188:dbl, "Load limit symmetry"=w187:enum32{"Symmetric", "Asymmetric"}, "Load current/voltage limit range"=w186:dbl, "Load current/voltage limit low"=w185:dbl, "Load current/voltage limit high"=w184:dbl, "Load output function"=w183:i32, "Load sense"=w182:i32, "Load transient response"=w181:i32, "Load voltage/current gain bandwidths"=w173:dbl[], "Load voltage/current compensation frequencies"=w172:dbl[], "Load voltage/current pole-zero ratios"=w171:dbl[])
        n43 = Unbundle By Name(w180) -> ("Load Master/Single resource name"=w191:string, "Load Slave resource name"=w190:string[])
        n44 = Index Array(array=w167, index=0) -> (element=w166:dbl)
        n45 = Index Array(array=w173, index=0) -> (element=w170:dbl)
        n46 = Index Array(array=w172, index=0) -> (element=w169:dbl)
        n47 = Index Array(array=w171, index=0) -> (element=w168:dbl)
        n48 = Bundle By Name(cluster=T7 {"Master resource name "="", "Slave resource names"=[], "System configuration"=enum."Parallel", "Voltage/current level"=0.0, "Voltage/current level range"=0.0, "Limit symmetry"=enum."Symmetric", "Voltage/current limit range"=0.0, "Voltage/current limit low"=0.0, "Voltage/current limit high"=inf, "Output function"=1007, "Sense"=1009, "Transient response"=1038, "Voltage/current gain bandwith"=0.0, "Voltage/current compensation frequency"=0.0, "Voltage/current pole-zero ratio"=0.0, "DUT set-up time"=0.0} ("Initialize Resource Config - Ganging"), "Master resource name"=w191, "Slave resource names"=w190, "DUT set-up time"=1.0, "System configuration"=w189, "Voltage/current level"=w166, "Voltage/current level range"=w188, "Limit symmetry"=w187, "Voltage/current limit range"=w186, "Voltage/current limit low"=w185, "Voltage/current limit high"=w184, "Output function"=w183, "Sense"=w182, "Transient response"=w181, "Voltage/current gain bandwith"=w170, "Voltage/current compensation frequency"=w169, "Voltage/current pole-zero ratio"=w168) -> (w194:T7)
        n49 = call "Initialize Resource Config-Ganging.vi"("error in"=w178, "Initialize Resource Config - Ganging"=w194) -> ("error out"=w163:errorcluster, "Ganged Session Out"=w193:T4)  [unwired: 8 in]
        n50 = Bundle By Name(cluster=w180, "Load Ganged Session Out"=w193) -> (w164:T3)
      }
      frame "InitializeLoadConfigurationSingle" {
        # "Initializing different properties for single load to set to single point"
        n51 = Unbundle By Name(w213) -> ("Load voltage/current setpoints"=w208:dbl[], "Load voltage/current level range"=w216:dbl, "Load limit symmetry"=w217:enum32{"Symmetric", "Asymmetric"}, "Load current/voltage limit range"=w218:dbl, "Load current/voltage limit low"=w219:dbl, "Load current/voltage limit high"=w220:dbl, "Load output function"=w221:i32, "Load sense"=w222:i32, "Load transient response"=w223:i32, "Load voltage/current gain bandwidths"=w202:dbl[], "Load voltage/current compensation frequencies"=w201:dbl[], "Load voltage/current pole-zero ratios"=w200:dbl[])
        n52 = Unbundle By Name(w212) -> ("Load Master/Single resource name"=w224:string)
        n53 = Index Array(array=w202, index=0) -> (element=w199:dbl)
        n54 = Index Array(array=w201, index=0) -> (element=w198:dbl)
        n55 = Index Array(array=w200, index=0) -> (element=w197:dbl)
        n56 = Index Array(array=w208, index=0) -> (element=w206:dbl)
        n57 = Bundle By Name(cluster=T8 {"Resource name"="", "Voltage/current level"=0.0, "Voltage/current level range"=0.0, "Voltage/current limit range"=0.0, "Voltage/current limit low"=0.0, "Voltage/current limit high"=inf, "Output function"=1007, "Sense"=1009, "Transient response"=1038, "Voltage/current gain bandwidth"=0.0, "Voltage/current compensation frequency"=0.0, "Voltage/current pole-zero ratio"=0.0, "DUT set-up time"=0.0, "Limit symmetry"=enum."Symmetric"} ("Initialize Resource Config - Single"), "Resource name"=w224, "DUT set-up time"=1.0, "Voltage/current level"=w206, "Voltage/current level range"=w216, "Limit symmetry"=w217, "Voltage/current limit range"=w218, "Voltage/current limit low"=w219, "Voltage/current limit high"=w220, "Output function"=w221, "Sense"=w222, "Transient response"=w223, "Voltage/current gain bandwidth"=w199, "Voltage/current compensation frequency"=w198, "Voltage/current pole-zero ratio"=w197) -> (w225:T8)
        n58 = call "Initialize Resource Config-Single.vi"("error in"=w211, "Initialize resource Config - Single"=w225) -> ("error out"=w196:errorcluster, "channel name"=w214:string, "instrument handle out"=w215:refnum<k15>)  [unwired: 7 in]
        n59 = Bundle By Name(cluster=w212, "Load session out"=w215, "Load channel name"=w214) -> (w209:T3)
      }
      frame "ConfigureSourceToSequenceGanged" {
        # "Configuring source ganged to sequence mode for different voltage/current and source delays"
        n60 = call "ConfigureSourcetoSequence-Ganged.vi"("error in"=w232, "measurement configuration"=w230, "Waveform Mode - Control"=w229) -> ("error out"=w228:errorcluster, "Waveform Mode - Results"=w231:T3)  [unwired: 7 in]
      }
      frame "ConfigureSourceToSequenceSingle" {
        # "Configuring source single to sequence mode for different voltage/current and source delays"
        n61 = call "Configure Source to Sequence - Single.vi"("error in"=w238, "measurement configuration"=w237, "Waveform Mode - Control"=w236) -> ("error out"=w234:errorcluster, "Waveform Mode - Result"=w235:T3)  [unwired: 7 in]
      }
      frame "ConfigureLoadToSequenceGanged" {
        # "Configuring load ganged to sequence mode for different voltage/current and source delays"
        n62 = call "Configure Load to Sequence - ganged.vi"("error in"=w244, "measurement configuration"=w242, "Waveform Mode - Control"=w241) -> ("error out"=w240:errorcluster, "Waveform Mode - Result"=w243:T3)  [unwired: 7 in]
      }
      frame "ConfigureLoadToSequenceSingle" {
        # "Configuring Load single to sequence mode for different voltage/current and source delays"
        n63 = call "Configure Load to Sequence - Single.vi"("error in"=w250, "measurement configuration"=w249, "Waveform Mode - Control"=w248) -> ("error out"=w247:errorcluster, "Waveform Mode - Results"=w245:T3)  [unwired: 7 in]
      }
      frame "StartAndInitiateOutput" {
        w266 = T10 1033 items=["Source Complete Event"=1030, "Measure Complete Event"=1031, "Sequence Iteration Complete Event"=1032, "Sequence Engine Done Event"=1033, "Pulse Complete Event"=1051, "Ready For Pulse Trigger Event"=1052] ("event")
        # "Start and initaite the output"
        n64 = Unbundle By Name(w254) -> ("Source Ganged Session Out"=w274:T4, "Load Ganged Session Out"=w273:T4, "Source session out"=w272:refnum<k15>, "Load session out"=w271:refnum<k15>, "Source channel name"=w270:string, "Load channel name"=w269:string, "Load ganged/single"=w268:bool, "Source ganged/single"=w267:bool, "Load Source ON/OFF"=w252:T16)
        n65 = Bundle By Name(cluster=T9 {"Source Ganged Session Out"={"Ganged Config"=enum."Series", "Session List"=[], "Session Mode"=[], "Channel"=[]}, "Load Ganged Session Out"={"Ganged Config"=enum."Series", "Session List"=[], "Session Mode"=[], "Channel"=[]}, "Source session out"="", "Load session out"="", "event"=1030, "Source channel name"="", "Load channel name"="", "Load Source ON/OFF"=enum."SOURCE AND LOAD OFF", "Load ganged/single"=FALSE, "Source ganged/single"=FALSE} ("Start and wait event config"), "Source Ganged Session Out"=w274, "Load Ganged Session Out"=w273, "Source session out"=w272, "Load session out"=w271, "Source channel name"=w270, "Load channel name"=w269, "Load ganged/single"=w268, "Source ganged/single"=w267, "Load Source ON/OFF"=w252, "event"=w266) -> (w257:T9)
        n66 = call "Start and Wait for Event.vi"("error in"=w256, "Start and wait event config"=w257) -> ("error out"=w255:errorcluster, "Start and wait event result"=w259:T9)  [unwired: 7 in]
        n67 = Unbundle By Name(w259) -> ("Source Ganged Session Out"=w265:T4, "Load Ganged Session Out"=w264:T4, "Source session out"=w263:refnum<k15>, "Load session out"=w262:refnum<k15>, "Source channel name"=w261:string, "Load channel name"=w260:string)
        n68 = Bundle By Name(cluster=w254, "Source Ganged Session Out"=w265, "Load Ganged Session Out"=w264, "Source session out"=w263, "Load session out"=w262, "Source channel name"=w261, "Load channel name"=w260) -> (w253:T3)
      }
      frame "PerformMeasurement" {
        # "Fetch the output for different configuration"
        n69 = call "Fetch Measurement - WaveformMode.vi"("error in"=w279, "Waveform Mode - Control"=w276) -> ("error out"=w277:errorcluster, "Waveform Mode - Result"=w278:T3)  [unwired: 8 in]
      }
      frame "AbortAndCloseSession" {
        # "Abort and closes session for different configuration"
        n70 = Unbundle By Name(w281) -> ("Load Source ON/OFF"=w290:T16, "Source ganged/single"=w288:bool, "Source First Sequence Call"=w284:bool, "Load ganged/single"=w289:bool, "Load First Sequence Call"=w283:bool)
        n71 = case shown="\"LOAD ON\"" w290 {
          tunnel: w288 -> [_ w298 _]
          tunnel: w281 -> [_ w297 w346]
          tunnel: w289 -> [_ _ w344]
          tunnel: [w292 w296 w345] -> w287
          tunnel: w282 -> [w292 w295 w347]
          tunnel: w284 -> [_ w294 _]
          tunnel: w283 -> [_ _ w343]
          tunnel: w281 -> [_ _ w338]
          tunnel: ["" "" w335] -> w280
          frame Default {
          }
          frame "SOURCE ON" {
            # "Source enable"
            n72 = case shown="True" w294 {
              tunnel: w298 -> [w302 w317]
              tunnel: w297 -> [w301 w318]
              tunnel: [w300 w316] -> w296
              tunnel: w295 -> [w299 w319]
              frame False {
                # "If Advance sequence is not called"
                n73 = case shown="False" w302 {
                  tunnel: w301 -> [w308 w315]
                  tunnel: [w304 w311] -> w300
                  tunnel: w299 -> [w305 w310]
                  frame False {
                    # "Ganged channel abort"
                    n74 = Unbundle By Name(w308) -> ("Source Ganged Session Out"=w306:T4)
                    n75 = Bundle By Name(cluster=T11 {"Ganged Session in"={"Ganged Config"=enum."Series", "Session List"=[], "Session Mode"=[], "Channel"=[]}} ("Ganged Session Out"), "Ganged Session in"=w306) -> (w303:T11)
                    n76 = call "Abort Single Point Source-Ganging.vi"("error in"=w305, "Ganged Session In"=w303) -> ("error out"=w304:errorcluster)  [unwired: 9 in]
                  }
                  frame True {
                    # "Single channel abort"
                    n77 = Unbundle By Name(w315) -> ("Source session out"=w314:refnum<k15>, "Source channel name"=w313:string)
                    n78 = Bundle By Name(cluster=T12 {"Resource out"="", "Resource channel name"=""} ("Abort Single Point - Single"), "Resource out"=w314, "Resource channel name"=w313) -> (w309:T12)
                    n79 = call "Abort Single Point Source-Single.vi"("error in"=w310, "Abort Single Point - Single"=w309) -> ("error out"=w311:errorcluster)  [unwired: 9 in]
                  }
                }
              }
              frame True {
                # "If Advance seqquence is called"
                n80 = case shown="True" w317 {
                  tunnel: w318 -> [w326 w334]
                  tunnel: [w320 w327] -> w316
                  tunnel: w319 -> [w321 w328]
                  frame False {
                    # "Ganged channel abort"
                    n81 = Unbundle By Name(w326) -> ("Source Ganged Session Out"=w325:T4, "Source Sequence Name"=w323:string)
                    n82 = Bundle By Name(cluster=T13 {"Ganged Session Out"={"Ganged Config"=enum."Series", "Session List"=[], "Session Mode"=[], "Channel"=[]}, "Sequence name"=""} ("Abort Sequence - Ganging"), "Ganged Session Out"=w325, "Sequence name"=w323) -> (w322:T13)
                    n83 = call "Abort Sequence Source-Ganging.vi"("error in"=w321, "Abort Sequence - Ganging"=w322) -> ("error out"=w320:errorcluster)  [unwired: 9 in]
                  }
                  frame True {
                    # "Single channel abort"
                    n84 = Unbundle By Name(w334) -> ("Source session out"=w333:refnum<k15>, "Source channel name"=w332:string, "Source Sequence Name"=w330:string)
                    n85 = Bundle By Name(cluster=T14 {"Resource out"="", "Resource channel name"="", "Source sequence name"=""} ("Abort Sequence - Single"), "Resource out"=w333, "Resource channel name"=w332, "Source sequence name"=w330) -> (w329:T14)
                    n86 = call "Abort Sequence Source-Single.vi"("error in"=w328, "Abort Sequence - Single"=w329) -> ("error out"=w327:errorcluster)  [unwired: 9 in]
                  }
                }
              }
            }
          }
          frame "LOAD ON" {
            # "Load enable"
            n87 = case shown="False" w343 {
              tunnel: w347 -> [w351 w366]
              tunnel: w346 -> [w350 w367]
              tunnel: [w349 w365] -> w345
              tunnel: w344 -> [w348 w368]
              frame False {
                # "If Advance seqquence is not called for load"
                n88 = case shown="False" w348 {
                  tunnel: w350 -> [w357 w364]
                  tunnel: [w353 w359] -> w349
                  tunnel: w351 -> [w354 w360]
                  frame False {
                    # "Ganged channel abort"
                    n89 = Unbundle By Name(w357) -> ("Source Ganged Session Out"=w355:T4)
                    n90 = Bundle By Name(cluster=T11 {"Ganged Session in"={"Ganged Config"=enum."Series", "Session List"=[], "Session Mode"=[], "Channel"=[]}} ("Ganged Session Out"), "Ganged Session in"=w355) -> (w352:T11)
                    n91 = call "Abort Single Point Load-Ganging.vi"("error in"=w354, "Ganged Session In"=w352) -> ("error out"=w353:errorcluster)  [unwired: 9 in]
                  }
                  frame True {
                    # "Single channel abort"
                    n92 = Unbundle By Name(w364) -> ("Load session out"=w363:refnum<k15>, "Load channel name"=w362:string)
                    n93 = Bundle By Name(cluster=T12 {"Resource out"="", "Resource channel name"=""} ("Abort Single Point - Single"), "Resource out"=w363, "Resource channel name"=w362) -> (w358:T12)
                    n94 = call "Abort Single Point Load-Single.vi"("error in"=w360, "Abort Single Point - Single"=w358) -> ("error out"=w359:errorcluster)  [unwired: 9 in]
                  }
                }
              }
              frame True {
                # "If Advance seqquence is called for load"
                n95 = case shown="False" w368 {
                  tunnel: w367 -> [w375 w383]
                  tunnel: [w370 w376] -> w365
                  tunnel: w366 -> [w371 w377]
                  frame False {
                    # "Ganged channel abort"
                    n96 = Unbundle By Name(w375) -> ("Load Ganged Session Out"=w374:T4, "Load Sequence Name"=w372:string)
                    n97 = Bundle By Name(cluster=T13 {"Ganged Session Out"={"Ganged Config"=enum."Series", "Session List"=[], "Session Mode"=[], "Channel"=[]}, "Sequence name"=""} ("Abort Sequence - Ganging"), "Ganged Session Out"=w374, "Sequence name"=w372) -> (w369:T13)
                    n98 = call "Abort Sequence-Load Ganging.vi"("error in"=w371, "Abort Sequence - Ganging"=w369) -> ("error out"=w370:errorcluster)  [unwired: 9 in]
                  }
                  frame True {
                    # "Single channel abort"
                    n99 = Unbundle By Name(w383) -> ("Load session out"=w382:refnum<k15>, "Load channel name"=w381:string, "Load Sequence Name"=w379:string)
                    n100 = Bundle By Name(cluster=T14 {"Resource out"="", "Resource channel name"="", "Source sequence name"=""} ("Abort Sequence - Single"), "Resource out"=w382, "Resource channel name"=w381, "Source sequence name"=w379) -> (w378:T14)
                    n101 = call "Abort Sequence Load-Single.vi"("error in"=w377, "Abort Sequence - Single"=w378) -> ("error out"=w376:errorcluster)  [unwired: 9 in]
                  }
                }
              }
            }
            n102 = Unbundle By Name(w338) -> ("No. of eload used"=w341:i32)
            n103 = Number To Decimal String(number=w341, width (-)=i16 3) -> (decimal integer string=w342:string)
            n104 = Concatenate Strings("NO. OF E-LOAD USED: ", w342) -> (w337:string)
            n105 = Select(t="", s=w345, f=w337) -> (s? t:f=w335:string)
          }
        }
        n106 = Bundle By Name(cluster=w281, "Measurement Results.Eload status"=w280) -> (w286:T3)
      }
      frame "Exit", Default {
        # "Stops the while loop and exit in case of error caused in queue"
      }
    }
  }
  "error out" <- w18
  "Measure Call Context out" <- w14
  n107 = Unbundle By Name(w15) -> ("Measurement Results"=→"Measurement Results":T1)
